vi "CAN BL Erase.vi"(6 "TimeOut":u32, 7 "FlashSize":u32, 9 "NodeAddr":u16, 10 "CANIndex":i32, 11 "DevHandle":i32) -> (3 "function return":i32)   [LabVIEW 2010, in "usb2can.lvlib"]
doc: "int WINAPI CAN_BL_Erase(int DevHandle,int CANIndex,unsigned short NodeAddr,unsigned int FlashSize,unsigned int TimeOut);"
uses:
  usb2can.lvlib
  USB2XXX.dll
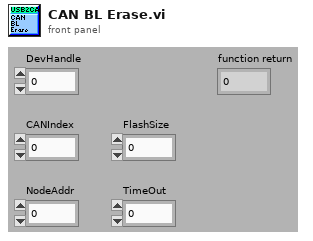
[diagram p1: front panel]
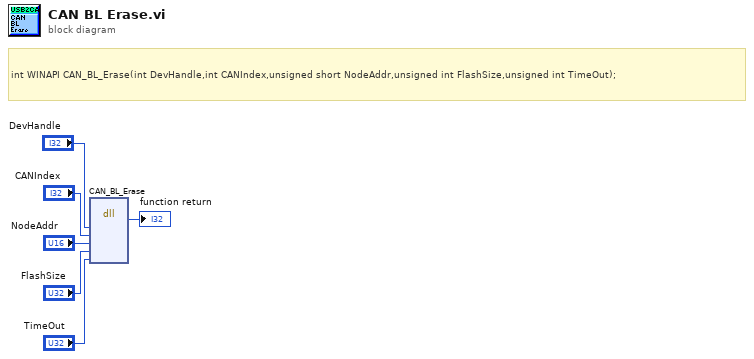
[diagram p0: block diagram]
diagram:
  # "int WINAPI CAN_BL_Erase(int DevHandle,int CANIndex,unsigned short NodeAddr,unsigned int FlashSize,unsigned int TimeOut);"
  n1 = dll-call lib="G:/OtherWork/USB2XXX_Example/trunk/Labview/PublicFiles/USB2XXX.*" fn="CAN_BL_Erase"("DevHandle"="DevHandle", "CANIndex"="CANIndex", "NodeAddr"="NodeAddr", "FlashSize"="FlashSize", "TimeOut"="TimeOut") -> (→"function return":i32)  [unwired: 8 in, 2 out]
